vi "Read Camera Name.vi"(8 "error in (no error)":errorcluster, 11 "HIJ Vision Camera App Dialog in":refnum<class "HIJ Vision Camera App Dialog.lvclass">) -> (0 "error out":errorcluster, 2 "IMAQdx Session":T1, 3 "HIJ Vision Camera App Dialog out":refnum<class "HIJ Vision Camera App Dialog.lvclass">)   [LabVIEW 2020, in "HIJ Vision Camera App Dialog.lvlib" / "HIJ Vision Camera App Dialog.lvclass"]
uses:
  HIJ Vision Camera App Dialog.lvclass
  HIJ Vision Camera App Dialog.lvclass/HIJ Vision Camera App Dialog.ctl
  <vilib>/userdefined/High Color/IMAQdx.ctl
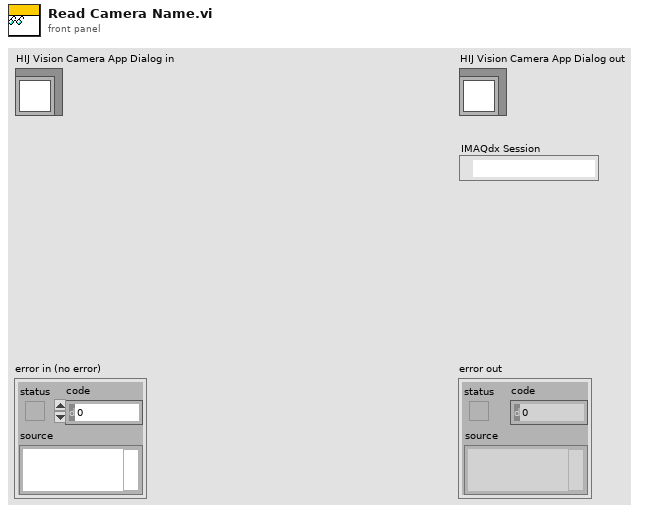
[diagram p1: front panel]
types:
  T1 = typedef "IMAQdx.ctl" = refnum<k21>
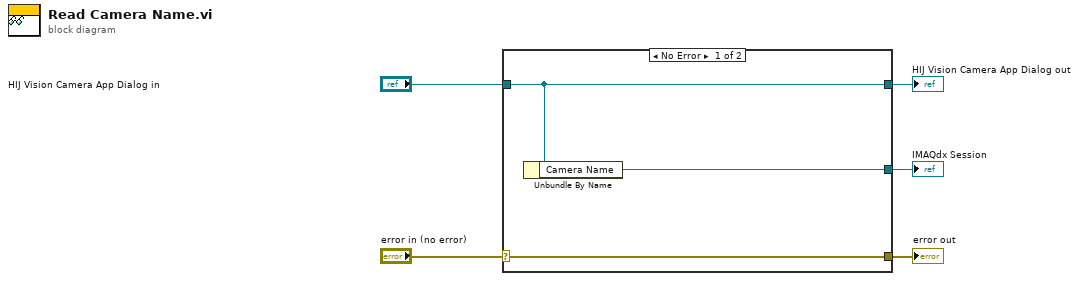
[diagram p0: block diagram]
diagram:
  n1 = case shown="No Error" "error in (no error)" {
    selector: "error in (no error)" -> [w8 w9]
    tunnel: [w8 w9] -> w4
    tunnel: [w7 w10] -> w2
    tunnel: "HIJ Vision Camera App Dialog in" -> [w7 w10]
    tunnel: [w6 _] -> w1
    frame No Error {
      n2 = Unbundle By Name(w7) -> ("Camera Name"=w6:T1)
    }
    frame Error {
    }
  }
  "error out" <- w4
  "HIJ Vision Camera App Dialog out" <- w2
  "IMAQdx Session" <- w1
